vi "TestExecuteOneShotSubscription_PublishOK.vi"(8 "error in (no error)":errorcluster, 11 "TestCase in":refnum<class "TestSubscriptionPolicy.lvclass">) -> (0 "error out":errorcluster, 3 "TestCase out":refnum<class "TestSubscriptionPolicy.lvclass">)   [LabVIEW 2020, in "TestSubscriptionPolicy.lvclass"]
uses:
  TestSubscriptionPolicy.lvclass
  TestSubscriptionPolicy.lvclass/TestSubscriptionPolicy.ctl
  Source/IMediator/ISubscriptionPolicy/ISubscriptionPolicy.lvclass
  Source/SubscriptionPolicy/OneShotSubscription/OneShotSubscription.lvclass
  modules/composed-transport/Source/Concrete/QueueTransport/QueueTransport.lvclass
  C:/Git/mva-core/modules/composed-transport/Source/ITransport/ITransport.lvclass
  C:/Git/mva-core/modules/composed-transport/Source/Concrete/QueueTransport/QueueTransport.lvclass
  C:/Git/mva-core/Source/IMediator/ISubscriptionPolicy/ISubscriptionPolicy.lvclass
  C:/Git/mva-core/Source/SubscriptionPolicy/OneShotSubscription/OneShotSubscription.lvclass
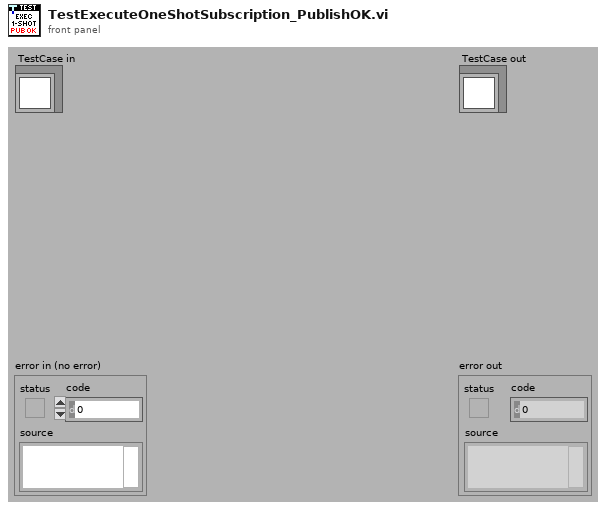
[diagram p1: front panel]
types:
  T1 = typedef "IMediator.lvlib/ISubscriptionPolicy.lvclass/ISubscriptionPolicy Reference.ctl" = refnum<data-value>
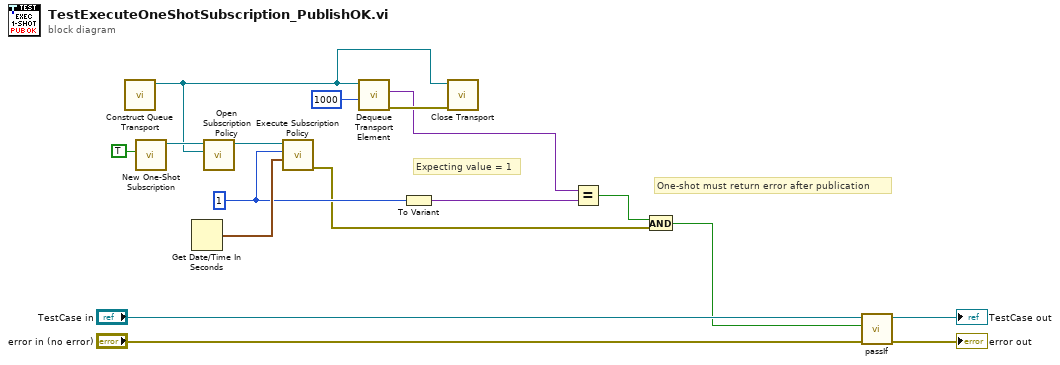
[diagram p0: block diagram]
diagram:
  w7 = 1
  # "One-shot must return error after publication"
  # "Expecting value = 1"
  n1 = call "Construct Queue Transport.vi"() -> ("QueueTransport"=w1:refnum<class "QueueTransport.lvclass">)  [unwired: 10 in, 1 out]
  n2 = call "New One-Shot Subscription.vi"("Ignore Past Updates? (F)"=TRUE) -> ("OneShotSubscription Out"=w9:refnum<class "OneShotSubscription.lvclass">)  [unwired: 10 in]
  n3 = Get Date/Time In Seconds() -> (seconds since 1Jan1904=w11:timestamp)
  n4 = call "Open Subscription Policy.vi"("Transport"=w1, "SubscriptionPolicy"=w9) -> ("Subscription Policy"=w13:T1)  [unwired: 8 in, 1 out]
  n5 = call "Execute Subscription Policy.vi"("Publish Time"=w11, "New Topic Value"=w7, "Subscription Policy"=w13) -> ("error out (Unsubscribe?)"=w4:errorcluster)  [unwired: 7 in, 1 out]
  n6 = call "Dequeue Transport Element.vi"("Timeout In ms (-1)"=1000, "QueueTransport"=w1) -> ("error out"=w10:errorcluster, "Data"=w2:variant)  [unwired: 6 in, 2 out]
  n7 = To Variant(anything=w7) -> (Variant=w6:variant)
  n8 = call-dynamic "Close Transport.vi"("error in (no error)"=w10, "QueueTransport"=w1) -> ()  [unwired: 9 in, 1 out]
  n9 = Equal?(x=w2, y=w6) -> (x = y?=w5:bool)
  n10 = And(x=w5, y=w4) -> (x .and. y?=w3:bool)
  n11 = call-dynamic "passIf.vi"("error in (no error)"="error in (no error)", "pass"=w3, "TestCase in"="TestCase in") -> ("error out"=→"error out":errorcluster, "TestCase out"=→"TestCase out":refnum<class "TestSubscriptionPolicy.lvclass">)  [unwired: 7 in]
